vi "GetTextInformation.vi"(8 "error in (no error)":errorcluster, 10 "Input":string, 11 "Code39 in":refnum<class "Code39.lvclass">) -> (0 "error out":errorcluster, 1 "Text":string, 2 "Text Positions":T1[](array[typedef]), 3 "Code39 out":refnum<class "Code39.lvclass">)   [LabVIEW 2013, in "BarCodes.lvlib" / "Code39.lvclass"]
doc: "Returns an array of clusters describing how text will be sized and positioned and the actual text to place below the bar code. The Start Index is the index in the returned string that each text info entry refers to. The length is the number of characters in the returned string that each text info entry refers to. The Text Rectangle is the rectangle to draw text in. The Clearing Rectangle is the rectangle to paint with the barcode's light color to make the text clear and visible. The font information is passed into the text writing function."
uses:
  Code39.lvclass
  BarCode/TextPosition.ctl
  BarCode/BarCode.lvclass
  BarCodes.lvlib
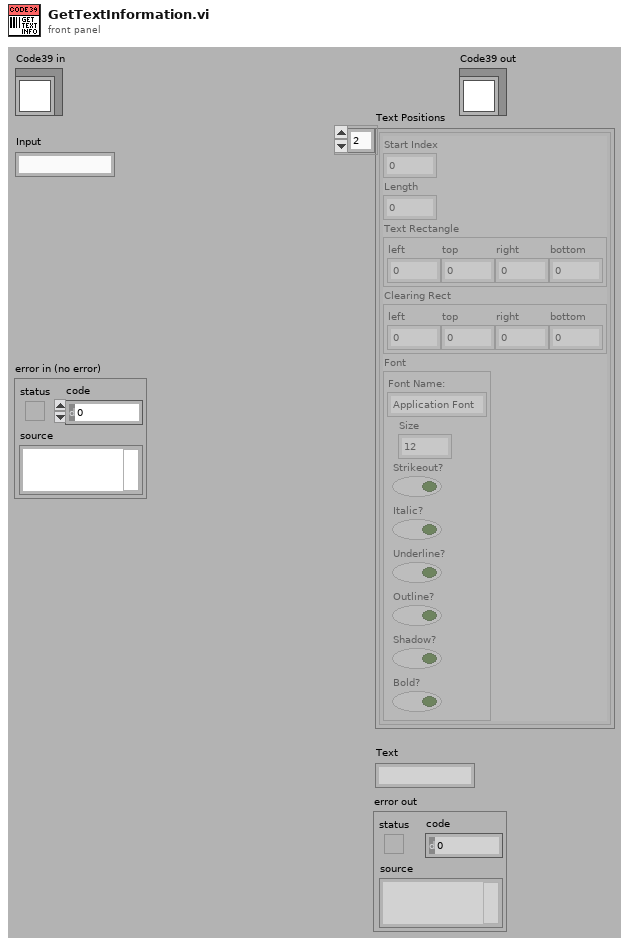
[diagram p1: front panel]
types:
  T1 = typedef "BarCodes.lvlib/BarCode.lvclass/TextPosition.ctl" = cluster{"Start Index":u8, "Length":u8, "Text Rectangle":cluster{"left":i16, "top":i16, "right":i16, "bottom":i16}, "Clearing Rect":cluster{"left":i16, "top":i16, "right":i16, "bottom":i16}, "Font":cluster{"Font Name:":string, "Size":i16, "Strikeout?":bool, "Italic?":bool, "Underline?":bool, "Outline?":bool, "Shadow?":bool, "Bold?":bool}}
  T2 = cluster{"left":i16, "top":i16, "right":i16, "bottom":i16}
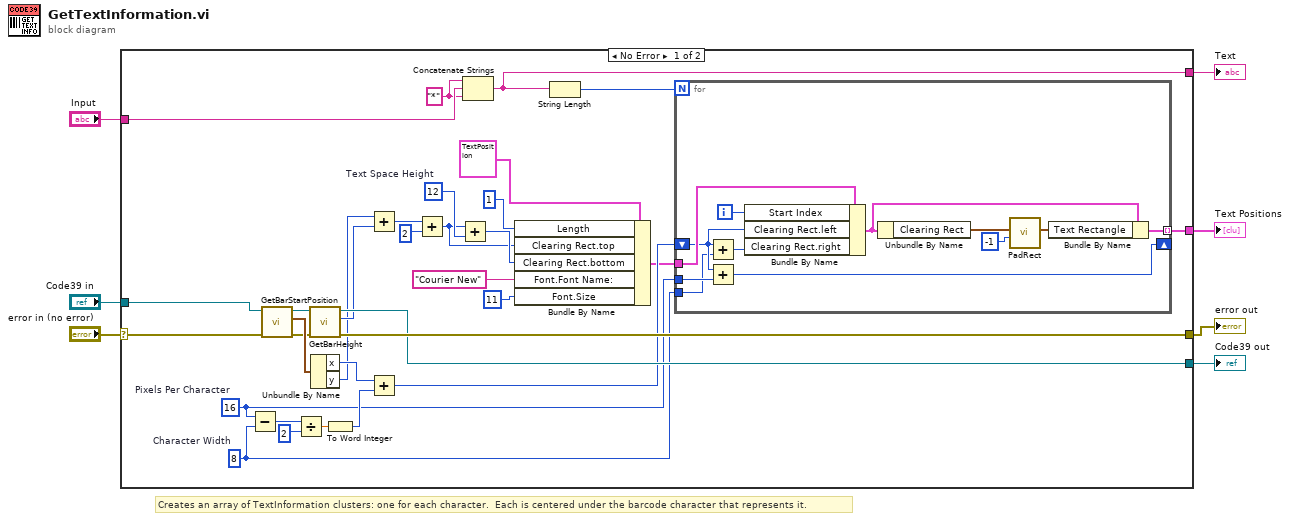
[diagram p0: block diagram]
diagram:
  # "Creates an array of TextInformation clusters: one for each character.  Each is centered under the barcode character that represents it."
  n1 = case shown="No Error" "error in (no error)" {
    selector: "error in (no error)" -> [w8 w52]
    tunnel: "Code39 in" -> [w39 w53]
    tunnel: [w35 w52] -> w6
    tunnel: [w34 w53] -> w5
    tunnel: "Input" -> [w32 w54]
    tunnel: [w24 w54] -> w3
    tunnel: [w13 _] -> w2
    frame No Error {
      w22 = i16 16  # Pixels Per Character
      w12 = i16 8  # Character Width
      w18 = i16 12  # Text Space Height
      w31 = "*" ("string")
      n2 = Subtract(x=w22, y=w12) -> (x-y=w30:i16)
      n3 = call-dynamic "GetBarStartPosition.vi"("error in (no error)"=w8, "Code39 in"=w39) -> ("error out"=w36:errorcluster, "Start Position"=w38:cluster{"x":i16, "y":i16}, "Code39 out"=w37:refnum<class "Code39.lvclass">)  [unwired: 7 in]
      n4 = Divide(x=w30, y=i16 2) -> (x/y=w28:dbl)
      n5 = call-dynamic "GetBarHeight.vi"("error in (no error)"=w36, "Code39 in"=w37) -> ("error out"=w35:errorcluster, "Bar Height"=w33:u8, "Code39 out"=w34:refnum<class "Code39.lvclass">)  [unwired: 7 in]
      n6 = Unbundle By Name(w38) -> ("x"=w27:i16, "y"=w11:i16)
      n7 = To Word Integer(number=w28) -> (16bit integer=w26:i16)
      n8 = Add(x=w11, y=w33) -> (x+y=w10:i16)
      n9 = Add(x=w27, y=w26) -> (x+y=w25:i16)
      n10 = Add(x=w10, y=i16 2) -> (x+y=w9:i16)
      n11 = Add(x=w9, y=w18) -> (x+y=w17:i16)
      n12 = Concatenate Strings(w31, w32, w31) -> (w24:string)
      n13 = Bundle By Name(cluster=T1 {"Start Index"=0, "Length"=0, "Text Rectangle"={"left"=0, "top"=0, "right"=0, "bottom"=0}, "Clearing Rect"={"left"=0, "top"=0, "right"=0, "bottom"=0}, "Font"={"Font Name:"="Application Font", "Size"=12, "Strikeout?"=FALSE, "Italic?"=FALSE, "Underline?"=FALSE, "Outline?"=FALSE, "Shadow?"=FALSE, "Bold?"=FALSE}} ("Text Position"), "Length"=u8 1, "Clearing Rect.top"=w9, "Clearing Rect.bottom"=w17, "Font.Font Name:"="Courier New", "Font.Size"=i16 11) -> (w14:T1)
      n14 = String Length(string=w24) -> (length=w23:i32)
      n15 = for {
        N: w23 -> [_]
        tunnel: w22 -> [w43]
        shift-right: [w41] -> _
        shift-left: w25 -> [w44]
        tunnel: w14 -> [w51]
        tunnel: [w46] -> w13 mode=indexing
        tunnel: w12 -> [w42]
        i -> [w40]
        n16 = Add(x=w44, y=w42) -> (x+y=w45:i16)
        n17 = Add(x=w44, y=w43) -> (x+y=w41:i16)
        n18 = Bundle By Name(cluster=w51, "Start Index"=w40, "Clearing Rect.left"=w44, "Clearing Rect.right"=w45) -> (w47:T1)
        n19 = Unbundle By Name(w47) -> ("Clearing Rect"=w50:T2)
        n20 = call "PadRect.vi"("Padding"=i8 -1, "Rectagle"=w50) -> ("Padded Rectangle"=w48:T2)  [unwired: 9 in]
        n21 = Bundle By Name(cluster=w47, "Text Rectangle"=w48) -> (w46:T1)
      }
    }
    frame Error {
    }
  }
  "error out" <- w6
  "Code39 out" <- w5
  "Text Positions" <- w2
  "Text" <- w3
